vi "Register Cluster.vi"(7 "Package Name":string, 8 "error in":errorcluster, 10 "Cluster":variant, 11 "gRPCid in":T1) -> (0 "error out":errorcluster, 3 "gRPCid out":T1)   [LabVIEW 2019, in "grpc-lvsupport.lvlib"]
uses:
  grpc-lvsupport.lvlib
  Shared/grpcId.ctl
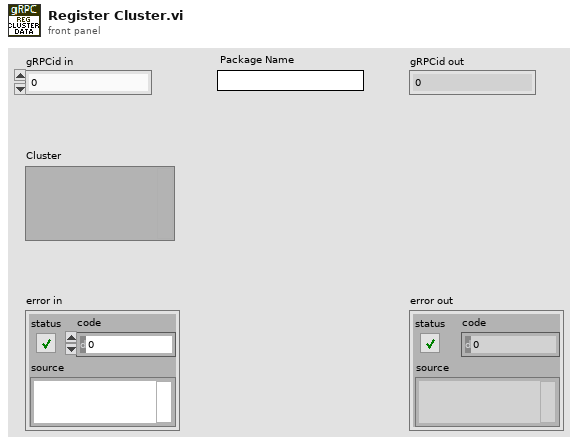
[diagram p1: front panel]
types:
  T1 = typedef "grpc-lvsupport.lvlib/grpcId.ctl" = u64
  T2 = typedef "gprc-lvsupport.lvlib/Message Metadata.ctl" = cluster{"Version":i32, "Name":string, "Type Url":string, "Elements":T3[]}
  T3 = typedef "gprc-lvsupport.lvlib/Message Element Metadata.ctl" = cluster{"Embedded Message Name":string, "Protobuf Index":i32, "MessageElementType":T4, "Repeated":bool}
  T4 = typedef "gprc-lvsupport.lvlib/Message Element Type.ctl" = enum32{"Int32Value", "FloatValue", "DoubleValue", "BoolValue", "StringValue", "MessageValue", "Int64Value", "UInt32Value", "UInt64Value", "EnumValue", "Bytes", "Fixed64", "Fixed32", "SFixed64", "SFixed32", "SInt64", "SInt32"}
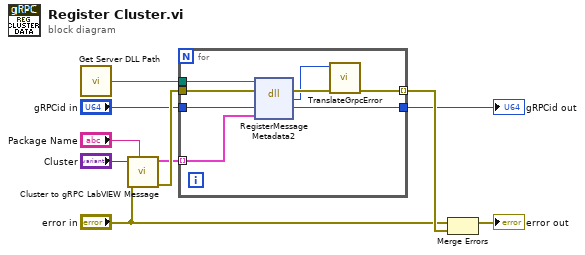
[diagram p0: block diagram]
diagram:
  n1 = call "Get Server DLL Path.vi"() -> ("Server dll path"=w6:path)
  n2 = call "Cluster to gRPC LabVIEW Message.vi"("Package Name"="Package Name", "error in"="error in", "Cluster"="Cluster") -> ("error out"=w9:errorcluster, "gRPC Message Metadata []"=w5:T2[])  [unwired: 7 in]
  n3 = for {
    tunnel: w5 -> [w16] mode=indexing
    tunnel: "gRPCid in" -> [w15]
    tunnel: w9 -> [w18]
    tunnel: [w12] -> w10 mode=indexing
    tunnel: [w14] -> w7
    tunnel: w6 -> [w13]
    n4 = dll-call lib="?" fn="RegisterMessageMetadata2"(path in=w13, error in=w18, "serverId"=w15, "metadata"=w16) -> (error out=w17:errorcluster, "return type"=w11:i32, "serverId"=w14:T1)  [unwired: 2 in, 1 out]
    n5 = call "TranslateGrpcError.vi"("error in"=w17, "Error Code"=w11) -> ("error out"=w12:errorcluster)  [unwired: 9 in]
  }
  "gRPCid out" <- w7
  n6 = Merge Errors("error in", w10) -> (→"error out":errorcluster)
